vi "CameraSimulationTester.vi"() -> ()   [LabVIEW 2017]
uses:
  Camera_Sim_class/Camera_Sim.lvclass
panel:
  in  "Simulated Image":path
  out "Connected":bool
  out "Frame Number":u32
  out "Image":T1(plugin-control)
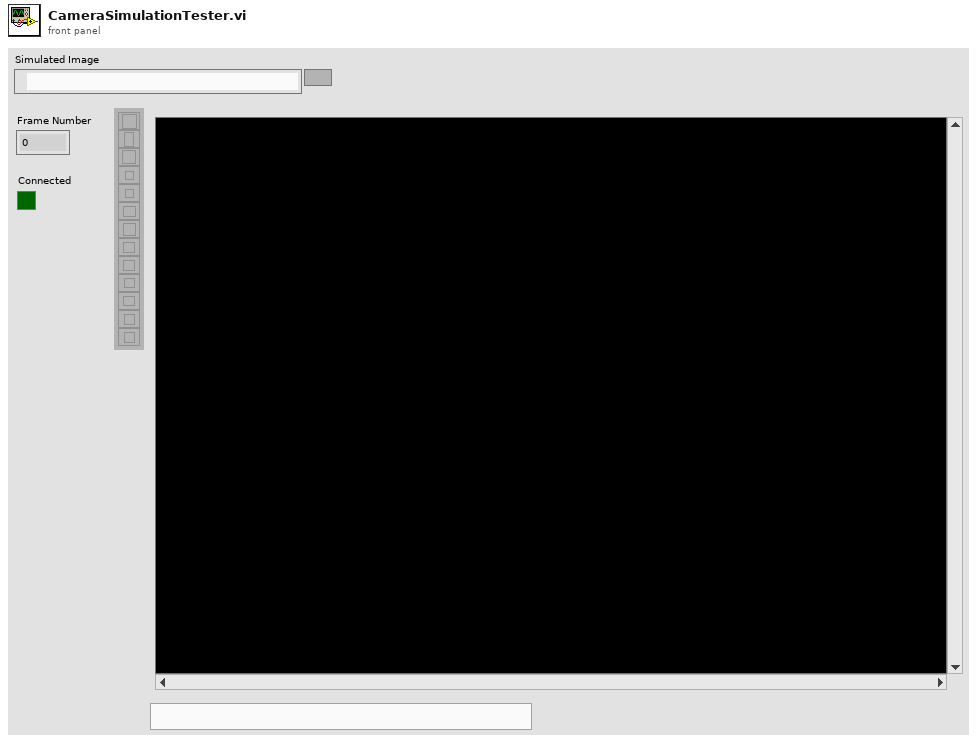
[diagram p1: front panel]
types:
  T1 = typedef "IMAQ Image.ctl" = refnum<image>
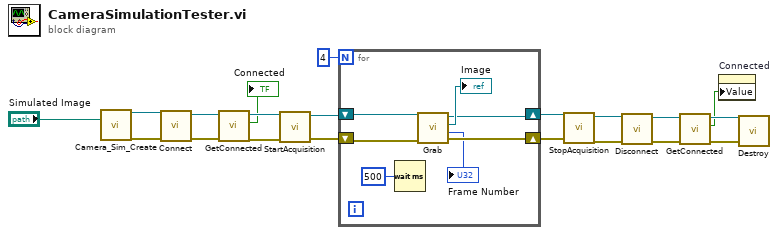
[diagram p0: block diagram]
diagram:
  n1 = call "Camera_Sim_Create.vi"("Simulated Image"="Simulated Image") -> ("reference out"=w19:refnum<class "Camera_Sim.lvclass">, "error out"=w18:errorcluster)  [unwired: 13 in]
  n2 = call-dynamic "Connect.vi"("error in (no error)"=w18, "reference in"=w19) -> ("error out"=w16:errorcluster, "reference out"=w17:refnum<class "Camera_Sim.lvclass">)  [unwired: 8 in]
  n3 = call-dynamic "GetConnected.vi"("error in (no error)"=w16, "reference in"=w17) -> ("error out"=w14:errorcluster, "Connected"=→"Connected":bool, "reference out"=w15:refnum<class "Camera_Sim.lvclass">)  [unwired: 7 in]
  n4 = call-dynamic "StartAcquisition.vi"("error in (no error)"=w14, "reference in"=w15) -> ("error out"=w12:errorcluster, "reference out"=w13:refnum<class "Camera_Sim.lvclass">)  [unwired: 8 in]
  n5 = for {
    N: 4 -> [_]
    shift-right: [w22] -> w10
    shift-left: w12 -> [w25]
    shift-right: [w23] -> w11
    shift-left: w13 -> [w26]
    n6 = Wait (ms)(milliseconds to wait=u32 500) -> ()  [unwired: 1 out]
    n7 = call-dynamic "Grab.vi"("error in (no error)"=w25, "reference in"=w26) -> ("error out"=w22:errorcluster, "Frame Number"=→"Frame Number":u32, "Image Out"=→"Image":T1, "reference out"=w23:refnum<class "Camera_Sim.lvclass">)  [unwired: 6 in]
  }
  n8 = call-dynamic "StopAcquisition.vi"("error in (no error)"=w10, "reference in"=w11) -> ("error out"=w8:errorcluster, "reference out"=w9:refnum<class "Camera_Sim.lvclass">)  [unwired: 8 in]
  n9 = call-dynamic "Disconnect.vi"("error in (no error)"=w8, "reference in"=w9) -> ("error out"=w5:errorcluster, "reference out"=w6:refnum<class "Camera_Sim.lvclass">)  [unwired: 8 in]
  n10 = call-dynamic "GetConnected.vi"("error in (no error)"=w5, "reference in"=w6) -> ("error out"=w3:errorcluster, "Connected"=w2:bool, "reference out"=w4:refnum<class "Camera_Sim.lvclass">)  [unwired: 7 in]
  n11 = property on="Connected" class="Bool (strict)"("Value"=w2) -> ()  [unwired: 2 in, 2 out]
  n12 = call-dynamic "Destroy.vi"("error in (no error)"=w3, "reference in"=w4) -> ()  [unwired: 8 in, 2 out]
